vi "Read OOB TX.vi"(8 "error in (no error)":errorcluster, 11 "CIFTemplatePlugin in":refnum<class "CIFTemplatePlugin.lvclass">) -> (0 "error out":errorcluster, 3 "CIFTemplatePlugin out":refnum<class "CIFTemplatePlugin.lvclass">)   [LabVIEW 2021, in "CIFTemplatePlugin.lvclass"]
uses:
  CIFTemplatePlugin.lvclass
  CIFTemplatePlugin.lvclass/CIFTemplatePlugin.ctl
  CIFUtilities/CIFOutOfBand/CIFOutOfBand.lvclass/CIFOutOfBand.ctl
  CIFUtilities/CIFOutOfBand/Read OOB DVR.vi
  OOB/OOB_Tx/Private/Command Settings.vi
  OOB/OOB_Tx/Private/Read Payload.vi
  CIFUtilities/CIFOutOfBand/Accessors/Read Local OOB Data.vi
  OOB/OOB_Tx/CIFCustomOOB_Tx.lvclass
  D:/dev/CIF-LVCore/src/CIFUtilities/CIFOutOfBand/CIFOutOfBand.lvclass
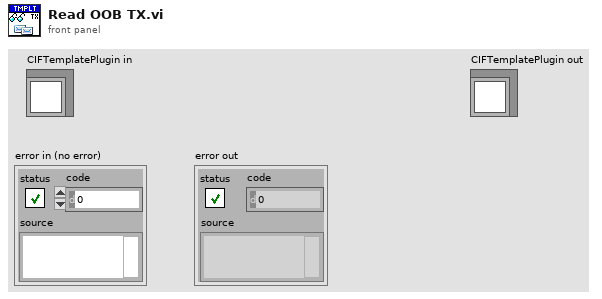
[diagram p1: front panel]
types:
  T1 = typedef "CIFCustomOOB_Tx.lvclass/OOB Commands.ctl" = enum8{"Update Data"}
  T2 = typedef "CIFCustomOOB_Tx.lvclass/Cyclic Data.ctl" = cluster{"Result":i32}
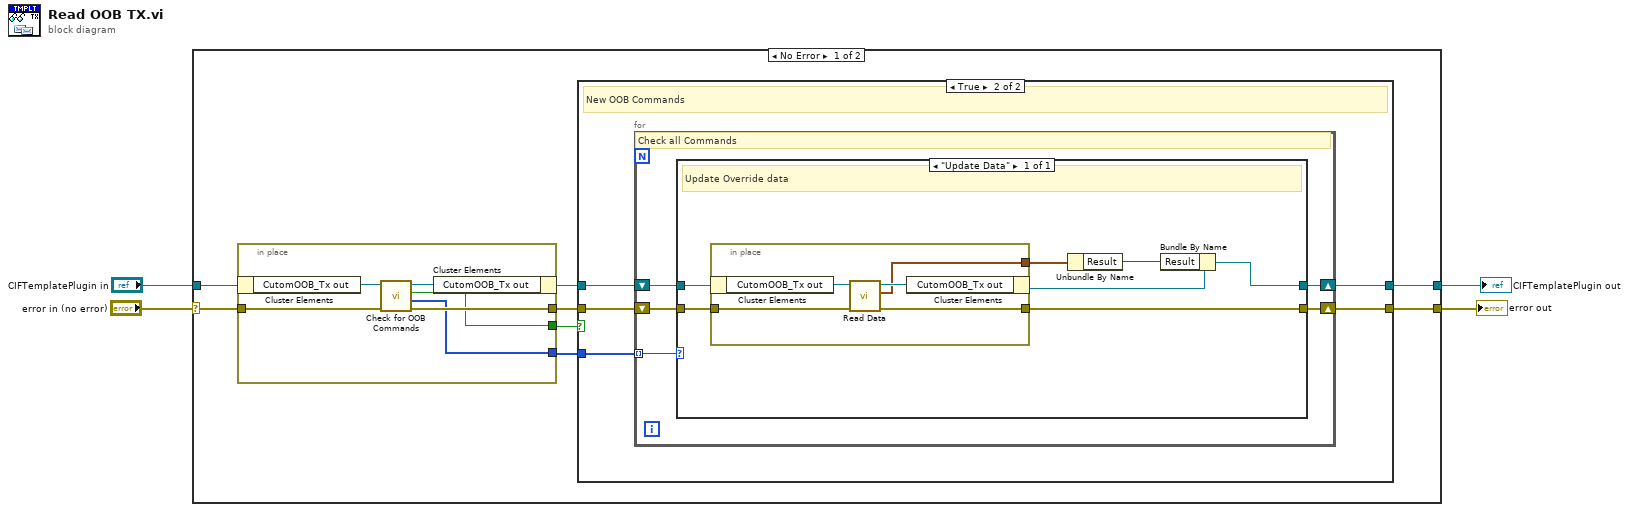
[diagram p0: block diagram]
diagram:
  n1 = case shown="No Error" "error in (no error)" {
    selector: "error in (no error)" -> [w11 w44]
    tunnel: [w5 w44] -> w3
    tunnel: [w7 w43] -> w1
    tunnel: "CIFTemplatePlugin in" -> [w12 w43]
    frame No Error {
      n2 = in-place {
        in-place-border: w11 -> [w41]
        in-place-border: [w39] -> w6
        in-place-border: [w38] -> w9
        in-place-border: [w37] -> w10
        n3 = in-place-cluster #1(w12) -> ("CutomOOB_Tx out"=w42:refnum<class "CIFCustomOOB_Tx.lvclass">)
        n4 = call "Check for OOB Commands.vi"("error in (no error)"=w41, "CutomOOB_Tx in"=w42) -> ("error out"=w39:errorcluster, "Commands"=w38:T1[], "New Commands"=w37:bool, "CutomOOB_Tx out"=w40:refnum<class "CIFCustomOOB_Tx.lvclass">)  [unwired: 6 in]
        n5 = in-place-cluster #1("CutomOOB_Tx out"=w40) -> (w8:refnum<class "CIFTemplatePlugin.lvclass">)
      }
      n6 = case shown="True" w10 {
        tunnel: w9 -> [_ w19]
        tunnel: w8 -> [w14 w18]
        tunnel: [w14 w16] -> w7
        tunnel: w6 -> [w13 w17]
        tunnel: [w13 w15] -> w5
        frame False {
          # "No new OOB Commands"
        }
        frame True {
          # "New OOB Commands"
          n7 = for {
            tunnel: w19 -> [w24] mode=indexing
            shift-right: [w21] -> w16
            shift-left: w18 -> [w22]
            shift-right: [w20] -> w15
            shift-left: w17 -> [w23]
            # "Check all Commands"
            n8 = case shown="\"Update Data\"" w24 {
              tunnel: w23 -> [w30]
              tunnel: w22 -> [w31]
              tunnel: [w25] -> w21
              tunnel: [w29] -> w20
              frame "Update Data" {
                # "Update Override data"
                n9 = in-place {
                  in-place-border: w30 -> [w35]
                  in-place-border: [w33] -> w29
                  in-place-border: [w32] -> w28
                  n10 = in-place-cluster #2(w31) -> ("CutomOOB_Tx out"=w36:refnum<class "CIFCustomOOB_Tx.lvclass">)
                  n11 = call "Read Data.vi"("error in"=w35, "CutomOOB_Tx in"=w36) -> ("error out"=w33:errorcluster, "Data"=w32:T2, "CutomOOB_Tx out"=w34:refnum<class "CIFCustomOOB_Tx.lvclass">)  [unwired: 7 in]
                  n12 = in-place-cluster #2("CutomOOB_Tx out"=w34) -> (w27:refnum<class "CIFTemplatePlugin.lvclass">)
                }
                n13 = Unbundle By Name(w28) -> ("Result"=w26:i32)
                n14 = Bundle By Name(cluster=w27, "Result"=w26) -> (w25:refnum<class "CIFTemplatePlugin.lvclass">)
              }
            }
          }
        }
      }
    }
    frame Error {
    }
  }
  "error out" <- w3
  "CIFTemplatePlugin out" <- w1
